vi "FusePose.vi"(0 "Vision Valid [t-?]":bool, 1 "Odometry Timestamp (ms)":u32, 2 "Odometry Delta X (in) [t0]":dbl, 3 "Odometry Delta Y (in) [t0]":dbl, 5 "Vision X (in) [t-?]":dbl, 7 "Vision Y (in) [t-?]":dbl, 9 "Vision Timestamp (ms)":u32, 12 "Pose Mode":T1(ring)) -> (4 "X (in) [t0]":dbl, 6 "Y (in) [t0]":dbl, 10 "X Odometry Only (in) [t0]":dbl, 15 "Y Odometry Only (in) [t0]":dbl)   [LabVIEW 2020]
doc: "This VI fuses multiple sensing modalities to estimate the robot's current pose."
uses:
  7b9bb9b1-306e-4d3e-b7ed-2eba6d8170c6.vi
  1559d662-8abd-40e9-a5dc-3c53134ee71a.vi
  524daecc-998c-4826-9d6e-2db19cf0bc7c.vi
  GlobalDriverStationData.vi
  GlobalDrivebase.vi
  GlobalPoseAndTargeting.vi
  GlobalDriverStationCommands.vi
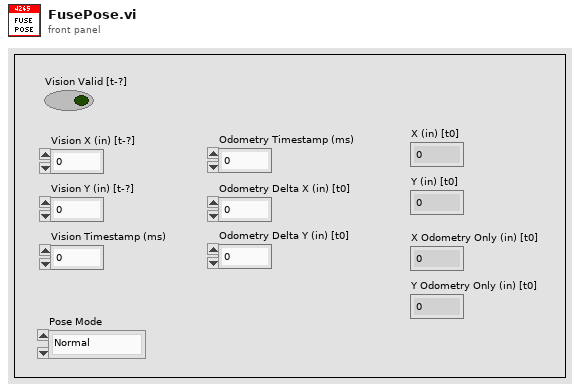
[diagram p1: front panel]
types:
  T1 = enum16{"Normal", "Auto Set", "Reset IMU", "Manual Push", "Init"}
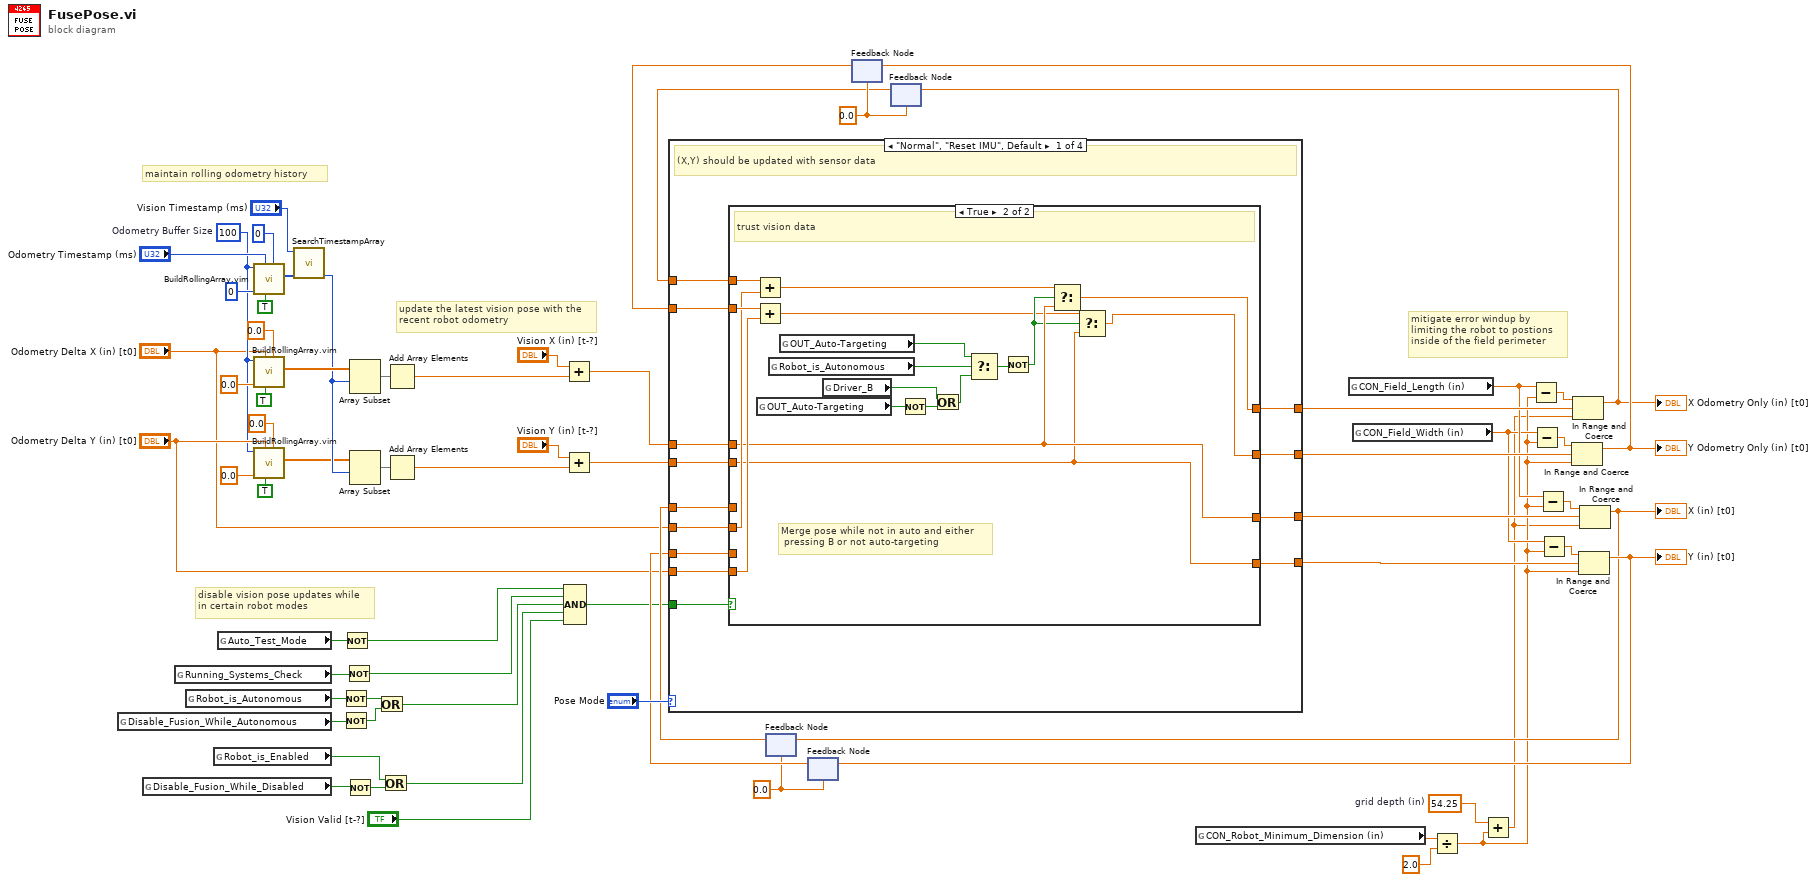
[diagram p0: block diagram]
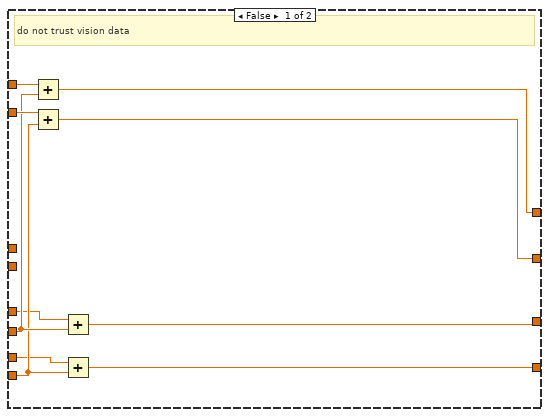
[diagram p2: hidden frame]
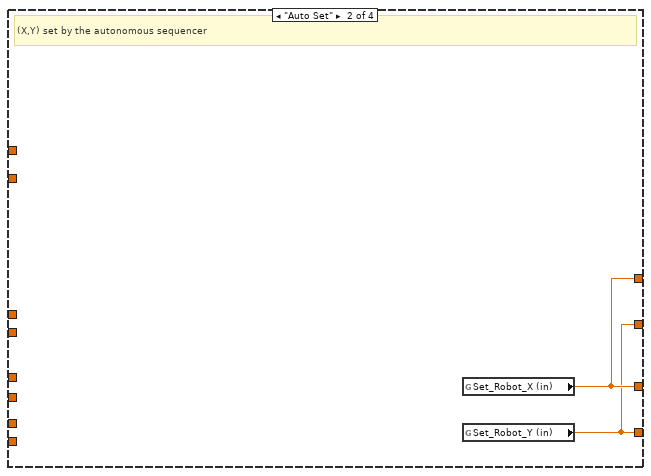
[diagram p3: hidden frame]
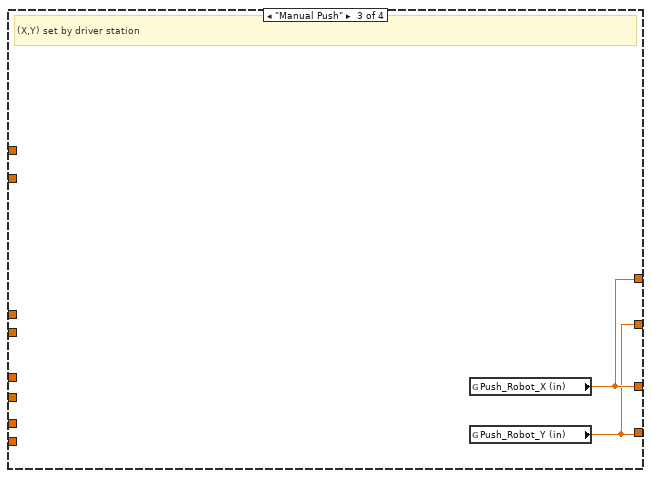
[diagram p4: hidden frame]
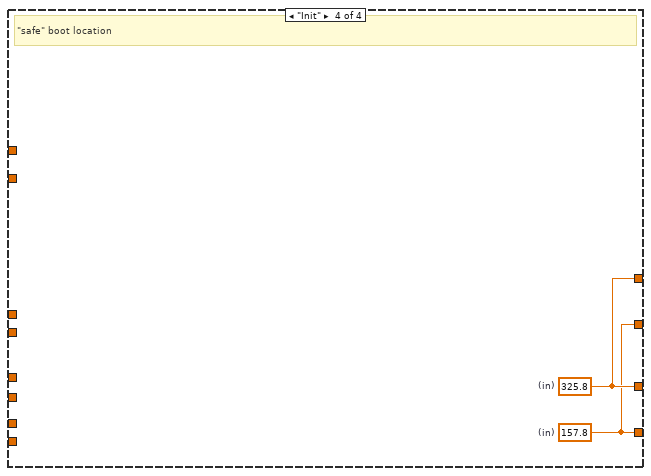
[diagram p5: hidden frame]
diagram:
  w5 = 54.25  # grid depth (in)
  w26 = 0.0
  w48 = 0.0
  w23 = 100  # Odometry Buffer Size
  # "disable vision pose updates while\nin certain robot modes"
  # "maintain rolling odometry history"
  # "update the latest vision pose with the\nrecent robot odometry"
  # "mitigate error windup by\nlimiting the robot to postions\ninside of the field perimeter"
  n1 = global read "GlobalDriverStationData.vi" "Disable_Fusion_While_Autonomous"() -> (w38:bool)
  n2 = global read "GlobalDriverStationData.vi" "Disable_Fusion_While_Disabled"() -> (w41:bool)
  n3 = global read "GlobalDriverStationData.vi" "Running_Systems_Check"() -> (w17:bool)
  n4 = global read "GlobalDriverStationData.vi" "Robot_is_Autonomous"() -> (w40:bool)
  n5 = global read "GlobalDriverStationData.vi" "Robot_is_Enabled"() -> (w6:bool)
  n6 = global read "GlobalDriverStationData.vi" "Auto_Test_Mode"() -> (w2:bool)
  n7 = call "BuildRollingArray.vim"("Global Additive Update"=0, "Update?"=TRUE, "New Value"="Odometry Timestamp (ms)", "Initial Value"=0, "Number of Elements"=w23) -> ("Current Array"=w63:u32[])  [unwired: 6 in]
  n8 = call "BuildRollingArray.vim"("Global Additive Update"=0.0, "Update?"=TRUE, "New Value"="Odometry Delta X (in) [t0]", "Initial Value"=0.0, "Number of Elements"=w23) -> ("Current Array"=w60:dbl[])  [unwired: 6 in]
  n9 = call "BuildRollingArray.vim"("Global Additive Update"=0.0, "Update?"=TRUE, "New Value"="Odometry Delta Y (in) [t0]", "Initial Value"=0.0, "Number of Elements"=w23) -> ("Current Array"=w55:dbl[])  [unwired: 6 in]
  n10 = call "SearchTimestampArray.vi"("Timestamp Array"=w63, "Search Timestamp"="Vision Timestamp (ms)") -> ("Closest Index"=w56:i32)  [unwired: 8 in, 1 out]
  n11 = Not(x=w40) -> (.not. x?=w39:bool)
  n12 = Not(x=w38) -> (.not. x?=w37:bool)
  n13 = Not(x=w2) -> (.not. x?=w1:bool)
  n14 = Not(x=w17) -> (.not. x?=w16:bool)
  n15 = Not(x=w41) -> (.not. x?=w35:bool)
  n16 = Array Subset(array=w60, index=w56) -> (w61:dbl[])  [unwired: 1 in]
  n17 = Array Subset(array=w55, index=w56) -> (w58:dbl[])  [unwired: 1 in]
  n18 = Or(x=w39, y=w37) -> (x .or. y?=w36:bool)
  n19 = Or(x=w6, y=w35) -> (x .or. y?=w34:bool)
  n20 = Add Array Elements(numeric array=w61) -> (sum=w59:dbl)
  n21 = Add Array Elements(numeric array=w58) -> (sum=w57:dbl)
  n22 = Add(x="Vision X (in) [t-?]", y=w59) -> (x+y=w52:dbl)
  n23 = Add(x="Vision Y (in) [t-?]", y=w57) -> (x+y=w53:dbl)
  n24 = Compound Arithmetic op=AND(w1, w16, w36, w34, "Vision Valid [t-?]") -> (w42:bool)
  n25 = feedback #1(w48) -> (w50:dbl)
  n26 = feedback #2(w48) -> (w49:dbl)
  n27 = feedback #3(w26) -> (w24:dbl)
  n28 = feedback #4(w26) -> (w25:dbl)
  n29 = case shown="\"Normal\", \"Reset IMU\", Default" "Pose Mode" {
    tunnel: [w76 w110 w112 w114] -> w11
    tunnel: w50 -> [w80 _ _ _]
    tunnel: "Odometry Delta X (in) [t0]" -> [w79 _ _ _]
    tunnel: w49 -> [w78 _ _ _]
    tunnel: "Odometry Delta Y (in) [t0]" -> [w77 _ _ _]
    tunnel: [w75 w109 w111 w113] -> w12
    tunnel: w42 -> [w74 _ _ _]
    tunnel: w53 -> [w73 _ _ _]
    tunnel: w52 -> [w72 _ _ _]
    tunnel: [w71 w110 w112 w114] -> w19
    tunnel: [w70 w109 w111 w113] -> w21
    tunnel: w25 -> [w69 _ _ _]
    tunnel: w24 -> [w68 _ _ _]
    frame "Normal", "Reset IMU", Default {
      # "(X,Y) should be updated with sensor data"
      n30 = case shown="True" w74 {
        tunnel: w80 -> [w84 _]
        tunnel: w79 -> [w86 w106]
        tunnel: w78 -> [w83 _]
        tunnel: w77 -> [w85 w105]
        tunnel: [w82 w99] -> w76
        tunnel: [w81 w97] -> w75
        tunnel: w73 -> [_ w97]
        tunnel: w72 -> [_ w99]
        tunnel: [w88 w101] -> w71
        tunnel: [w87 w95] -> w70
        tunnel: w69 -> [w90 w108]
        tunnel: w68 -> [w89 w107]
        frame False {
          # "do not trust vision data"
          n31 = Add(x=w90, y=w86) -> (x+y=w88:dbl)
          n32 = Add(x=w89, y=w85) -> (x+y=w87:dbl)
          n33 = Add(x=w84, y=w86) -> (x+y=w82:dbl)
          n34 = Add(x=w83, y=w85) -> (x+y=w81:dbl)
        }
        frame True {
          # "Merge pose while not in auto and either\n pressing B or not auto-targeting"
          # "trust vision data"
          n35 = Add(x=w108, y=w106) -> (x+y=w100:dbl)
          n36 = Add(x=w107, y=w105) -> (x+y=w96:dbl)
          n37 = global read "GlobalDrivebase.vi" "OUT_Auto-Targeting"() -> (w104:bool)
          n38 = global read "GlobalDriverStationData.vi" "Robot_is_Autonomous"() -> (w94:bool)
          n39 = global read "GlobalDrivebase.vi" "OUT_Auto-Targeting"() -> (w91:bool)
          n40 = global read "GlobalDriverStationCommands.vi" "Driver_B"() -> (w103:bool)
          n41 = Not(x=w104) -> (.not. x?=w102:bool)
          n42 = Or(x=w103, y=w102) -> (x .or. y?=w93:bool)
          n43 = Select(t=w91, s=w94, f=w93) -> (s? t:f=w92:bool)
          n44 = Not(x=w92) -> (.not. x?=w98:bool)
          n45 = Select(t=w100, s=w98, f=w99) -> (s? t:f=w101:dbl)
          n46 = Select(t=w96, s=w98, f=w97) -> (s? t:f=w95:dbl)
        }
      }
    }
    frame "Auto Set" {
      # "(X,Y) set by the autonomous sequencer"
      n47 = global read "GlobalPoseAndTargeting.vi" "Set_Robot_X (in)"() -> (w110:dbl)
      n48 = global read "GlobalPoseAndTargeting.vi" "Set_Robot_Y (in)"() -> (w109:dbl)
    }
    frame "Manual Push" {
      # "(X,Y) set by driver station"
      n49 = global read "GlobalPoseAndTargeting.vi" "Push_Robot_X (in)"() -> (w112:dbl)
      n50 = global read "GlobalPoseAndTargeting.vi" "Push_Robot_Y (in)"() -> (w111:dbl)
    }
    frame "Init" {
      w113 = 157.8  # (in)
      w114 = 325.8  # (in)
      # "\"safe\" boot location"
    }
  }
  n51 = global read "GlobalDrivebase.vi" "CON_Robot_Minimum_Dimension (in)"() -> (w15:dbl)
  n52 = global read "GlobalPoseAndTargeting.vi" "CON_Field_Length (in)"() -> (w10:dbl)
  n53 = global read "GlobalPoseAndTargeting.vi" "CON_Field_Width (in)"() -> (w9:dbl)
  n54 = Divide(x=w15, y=2.0) -> (x/y=w4:dbl)
  n55 = Add(x=w5, y=w4) -> (x+y=w3:dbl)
  n56 = Subtract(x=w10, y=w4) -> (x-y=w27:dbl)
  n57 = Subtract(x=w9, y=w4) -> (x-y=w28:dbl)
  n58 = Subtract(x=w10, y=w4) -> (x-y=w13:dbl)
  n59 = Subtract(x=w9, y=w4) -> (x-y=w14:dbl)
  n60 = In Range and Coerce(upper limit=w28, x=w21, lower limit=w4) -> (coerced(x)=w20:dbl)  [unwired: 1 out]
  "Y Odometry Only (in) [t0]" <- w20
  n61 = feedback-in #3(w20) -> ()
  n62 = In Range and Coerce(upper limit=w27, x=w19, lower limit=w3) -> (coerced(x)=w18:dbl)  [unwired: 1 out]
  "X Odometry Only (in) [t0]" <- w18
  n63 = feedback-in #4(w18) -> ()
  n64 = In Range and Coerce(upper limit=w14, x=w12, lower limit=w4) -> (coerced(x)=w8:dbl)  [unwired: 1 out]
  "Y (in) [t0]" <- w8
  n65 = feedback-in #2(w8) -> ()
  n66 = In Range and Coerce(upper limit=w13, x=w11, lower limit=w3) -> (coerced(x)=w7:dbl)  [unwired: 1 out]
  "X (in) [t0]" <- w7
  n67 = feedback-in #1(w7) -> ()
